vi "VelocityCommand.vi"(4 "PID gains Vel D":cluster{"(Kp)":dbl, "(Ki)":dbl, "(Kd)":dbl}={"(Kp)"=0.0, "(Ki)"=0.3, "(Kd)"=1.0}, 5 "intervalo":dbl=0.016, 6 "output xy":dbl format="%#_13g", 7 "estimatives":T1, 8 "Velocities Y":dbl[](array[numeric]), 9 "Time Y":dbl[](array[numeric]), 10 "Velocities X":dbl[](array[numeric]), 11 "Time X":dbl[](array[numeric])) -> (1 "Vy":dbl, 2 "Vx":dbl)   [LabVIEW 2018]
uses:
  <vilib>/Analysis/_algsub.llb/Real Vector Norm.vi
  <vilib>/Analysis/NI_AALPro.lvlib
panel:
  in  "size error array":i32=20
  out "Velocity Profile Y":cluster{"Time Y":dbl[], "Velocities Y":dbl[]}[](graph)
  out "Velocity Profile X":cluster{dbl[], dbl[]}[](graph)
  in  "est_vx":dbl
  in  "est_vy":dbl
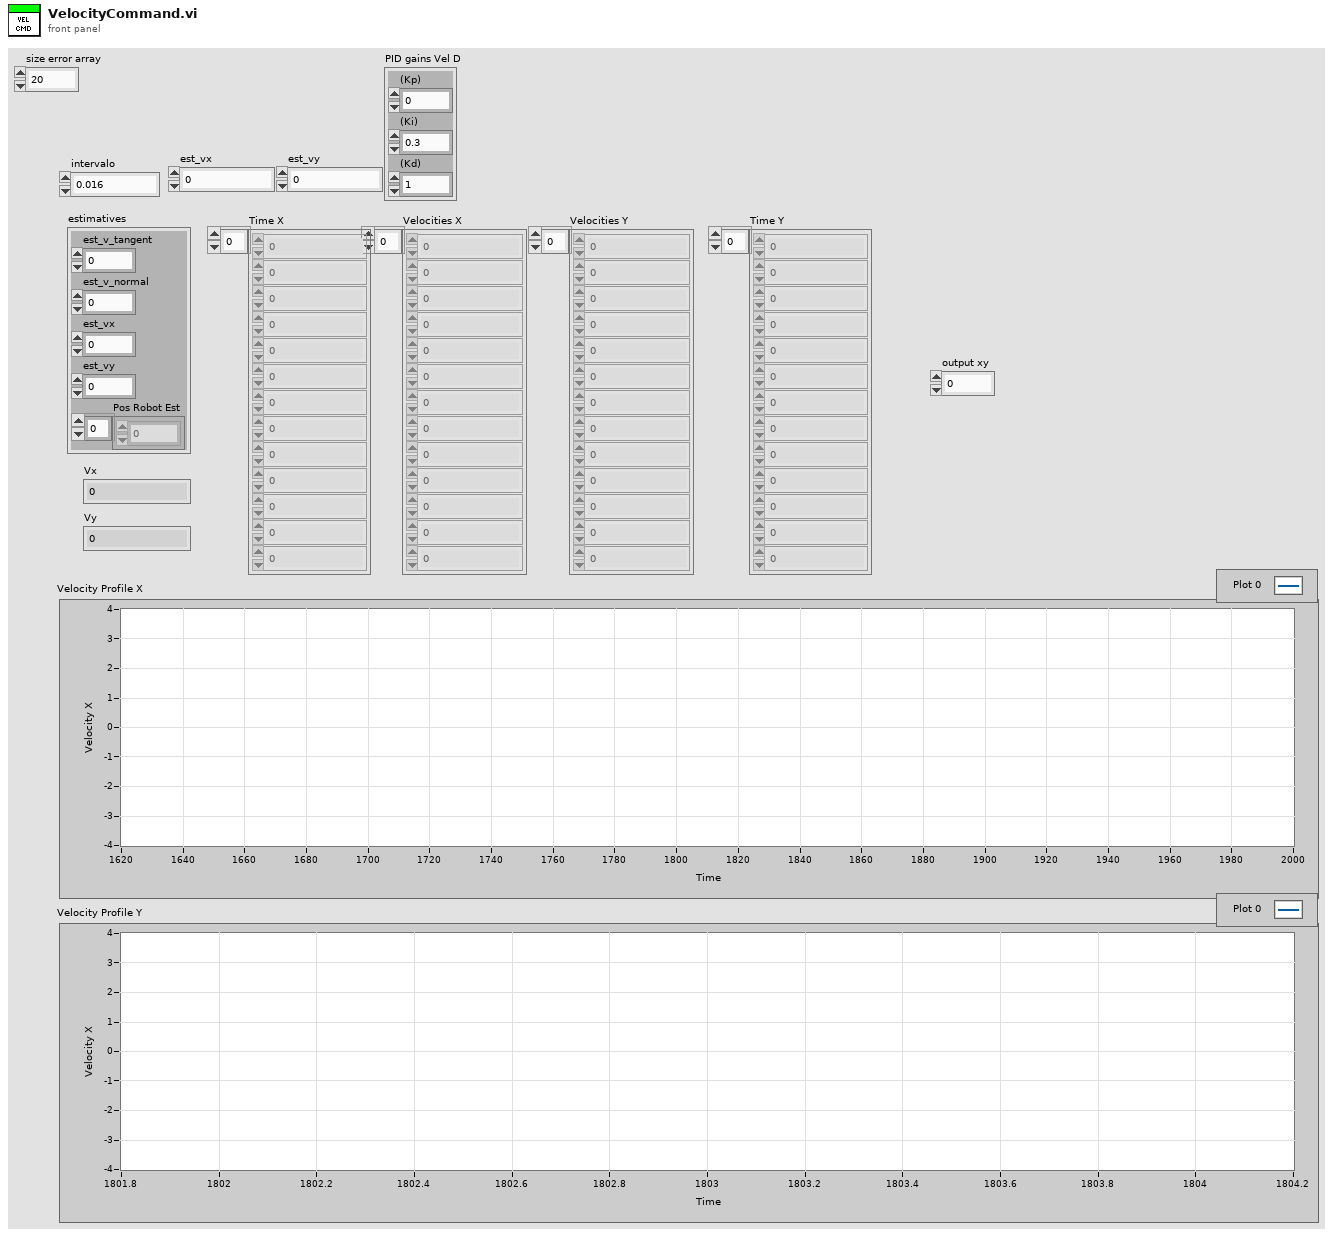
[diagram p1: front panel]
types:
  T1 = cluster{"est_v_tangent":dbl, "est_v_normal":dbl, "est_vx":dbl, "est_vy":dbl, "Pos Robot Est":dbl[]}
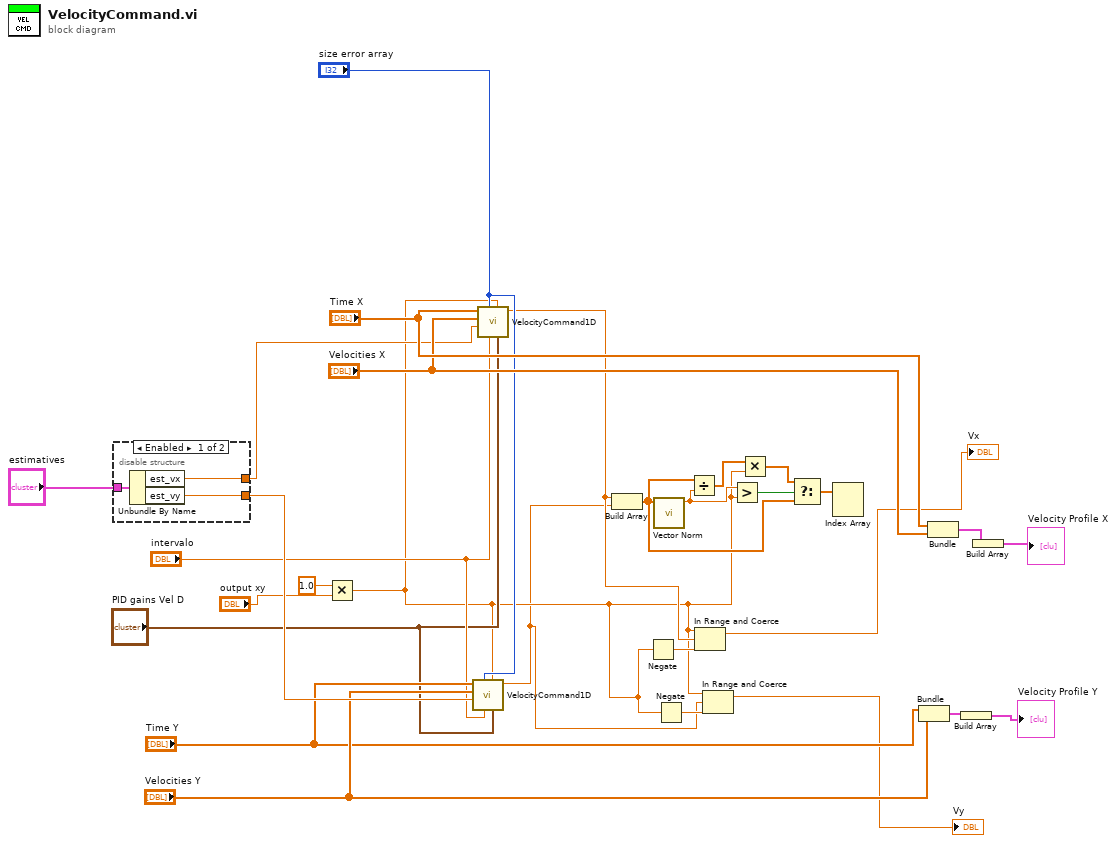
[diagram p0: block diagram]
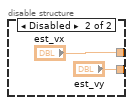
[diagram p2: hidden frame]
diagram:
  n1 = disable-structure shown="Enabled" {
    disable-tunnel: "estimatives" -> [w32 _]
    disable-tunnel: [w31 "est_vx"] -> w23
    disable-tunnel: [w30 "est_vy"] -> w15
    frame Enabled {
      n2 = Unbundle By Name(w32) -> ("est_vx"=w31:dbl, "est_vy"=w30:dbl)
    }
    frame Disabled {
    }
  }
  n3 = Multiply(x=1.0, y="output xy") -> (x*y=w4:dbl)
  n4 = call "VelocityCommand1D.vi"("PID gains Vel D"="PID gains Vel D", "output xy"=w4, "intervalo"="intervalo", "size error array"="size error array", "est_v"=w15, "Velocities"="Velocities Y", "Time"="Time Y") -> ("uk"=w1:dbl)  [unwired: 4 in]
  n5 = call "VelocityCommand1D.vi"("PID gains Vel D"="PID gains Vel D", "output xy"=w4, "intervalo"="intervalo", "size error array"="size error array", "est_v"=w23, "Velocities"="Velocities X", "Time"="Time X") -> ("uk"=w6:dbl)  [unwired: 4 in]
  n6 = Build Array(w6, w1) -> (w21:dbl[])
  n7 = Negate(x=w4) -> (-x=w7:dbl)
  n8 = call-poly <vilib>:"Vector Norm.vi"("Input Vector"=w21) -> ("norm"=w18:dbl)  [unwired: 9 in, 1 out]
  n9 = Negate(x=w4) -> (-x=w5:dbl)
  n10 = Divide(x=w21, y=w18) -> (x/y=w22:dbl[])
  n11 = In Range and Coerce(upper limit=w4, x=w6, lower limit=w7) -> (coerced(x)=→"Vx":dbl)  [unwired: 1 out]
  n12 = In Range and Coerce(upper limit=w4, x=w1, lower limit=w5) -> (coerced(x)=→"Vy":dbl)  [unwired: 1 out]
  n13 = Greater?(x=w18, y=w4) -> (0:w19:bool)
  n14 = Multiply(x=w22, y=w4) -> (x*y=w20:dbl[])
  n15 = Select(t=w20, s=w19, f=w21) -> (s? t:f=w17:dbl[])
  n16 = Index Array(array=w17) -> ()  [unwired: 2 in, 2 out]
  n17 = Bundle("Time Y"="Time Y", "Velocities Y"="Velocities Y") -> (w25:cluster{"Time Y":dbl[], "Velocities Y":dbl[]})  [unwired: 1 in]
  n18 = Bundle("Time X"="Time X", "Velocities X"="Velocities X") -> (w28:cluster{"Time X":dbl[], "Velocities X":dbl[]})  [unwired: 1 in]
  n19 = Build Array(w25) -> (→"Velocity Profile Y":cluster{"Time Y":dbl[], "Velocities Y":dbl[]}[])
  n20 = Build Array(w28) -> (→"Velocity Profile X":cluster{"Time X":dbl[], "Velocities X":dbl[]}[])
